vi "Update Project Symbol.vi"(8 "error in (no error)":errorcluster, 10 "New FPGA Personality Value":string, 11 "TargetItem Refnum":refnum<vi>) -> (0 "error out":errorcluster, 3 "Duplicated TargetItem Refnum":refnum<vi>)   [LabVIEW 2021, in "Personality.lvlib"]
doc: "Updates the FPGA personality disable symbol value with the new value."
uses:
  <vilib>/myRIO/Common/FPGA Personality Framework/Personality.lvlib
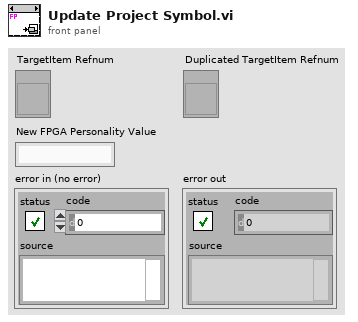
[diagram p1: front panel]
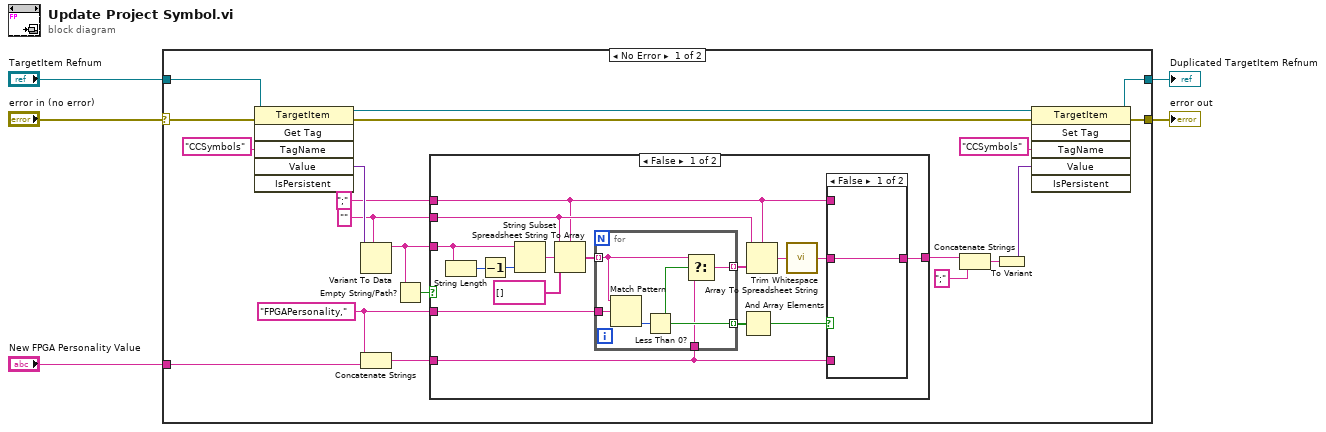
[diagram p0: block diagram]
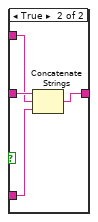
[diagram p2: hidden frame]
diagram:
  n1 = case shown="No Error" "error in (no error)" {
    selector: "error in (no error)" -> [w8 w55]
    tunnel: "New FPGA Personality Value" -> [w17 _]
    tunnel: "TargetItem Refnum" -> [w10 w54]
    tunnel: [w6 w54] -> w3
    tunnel: [w7 w55] -> w1
    frame No Error {
      w18 = "FPGAPersonality," ("regular expression")
      w21 = ""
      n2 = invoke class="TargetItem" method="Get Tag"(reference=w10, error in=w8, "TagName"="CCSymbols" ("Tag Name")) -> (reference out=w12:refnum<vi>, error out=w9:errorcluster, "Value"=w24:variant)  [unwired: 3 in, 3 out]
      n3 = Variant To Data(type=w21, Variant=w24) -> (data=w22:string)  [unwired: 1 in, 1 out]
      n4 = Concatenate Strings(w18, w17) -> (w19:string)
      n5 = Empty String/Path?(string/path=w22) -> (empty?=w23:bool)
      n6 = case shown="False" w23 {
        tunnel: w22 -> [w39 _]
        tunnel: w21 -> [w33 _]
        tunnel: ";" ("delimiter (Tab)") -> [w29 _]
        tunnel: w18 -> [w35 _]
        tunnel: w19 -> [w28 w53]
        tunnel: [w27 w53] -> w16
        frame False {
          n7 = String Length(string=w39) -> (length=w41:i32)
          n8 = Decrement(x=w41) -> (x-1=w40:i32)
          n9 = String Subset(string=w39, length (rest)=w40) -> (substring=w38:string)  [unwired: 1 in]
          n10 = Spreadsheet String To Array(delimiter (Tab)=w29, format string=w33, spreadsheet string=w38, array type (2D Dbl)=string[] []) -> (array=w36:string[])
          n11 = for {
            tunnel: w36 -> [w50] mode=indexing
            tunnel: w35 -> [w52]
            tunnel: [w49] -> w34 mode=indexing
            tunnel: [w48] -> w32 mode=indexing
            tunnel: w28 -> [w47]
            n12 = Match Pattern(string=w50, regular expression=w52) -> (offset past match=w51:i32)  [unwired: 1 in, 3 out]
            n13 = Less Than 0?(x=w51) -> (x < 0?=w48:bool)
            n14 = Select(t=w50, s=w48, f=w47) -> (s? t:f=w49:string)
          }
          n15 = And Array Elements(Boolean array=w32) -> (logical AND=w31:bool)
          n16 = Array To Spreadsheet String(delimiter (Tab)=w29, array=w34, 3:w33) -> (spreadsheet string=w30:string)
          n17 = call <vilib>:"Trim Whitespace.vi"("string"=w30) -> ("trimmed string"=w26:string)  [unwired: 1 in]
          n18 = case shown="False" w31 {
            tunnel: w26 -> [w42 w46]
            tunnel: [w42 w45] -> w27
            tunnel: w29 -> [_ w44]
            tunnel: w28 -> [_ w43]
            frame False {
            }
            frame True {
              n19 = Concatenate Strings(w46, w44, w43) -> (w45:string)
            }
          }
        }
        frame True {
        }
      }
      n20 = Concatenate Strings(w16, ";") -> (w14:string)
      n21 = To Variant(anything=w14) -> (Variant=w13:variant)
      n22 = invoke class="TargetItem" method="Set Tag"(reference=w12, error in=w9, "TagName"="CCSymbols" ("Tag Name"), "Value"=w13) -> (reference out=w6:refnum<vi>, error out=w7:errorcluster)  [unwired: 2 in, 4 out]
    }
    frame Error {
    }
  }
  "error out" <- w1
  "Duplicated TargetItem Refnum" <- w3
